vi "Within Msgs.vi"(9 "Msg":refnum<class "Msg.lvclass">, 10 "Msgs":T1) -> (2 "Within Msgs":bool)   [LabVIEW 2020, in "jettl.lvlib"]
uses:
  jettl.lvlib
  Msg/Msg.lvclass
  Msgs.ctl
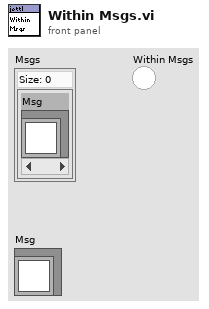
[diagram p1: front panel]
types:
  T1 = typedef "jettl.lvlib/Msgs.ctl" = set{refnum<class "Msg.lvclass">}
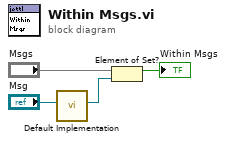
[diagram p0: block diagram]
diagram:
  n1 = call "Default Implementation.vi"("Implementation"="Msg") -> ("Default Implementation"=w1:refnum<class "Msg.lvclass">)  [unwired: 10 in]
  n2 = Element of Set?(10:w1, 11:"Msgs") -> (3:→"Within Msgs":bool)
